vi "3-6For循环的使用(下).vi"() -> ()   [LabVIEW 2018]
panel:
  out "字符串":string
  # "找到10000内的完数。完数指一个数恰好等于它本身的因子之和，例如28=14+7+4+2+1，6=3+2+1。"
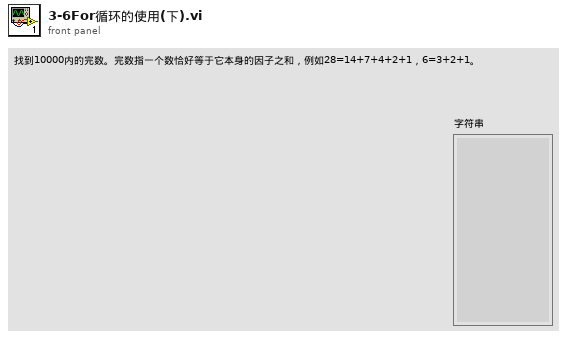
[diagram p1: front panel]
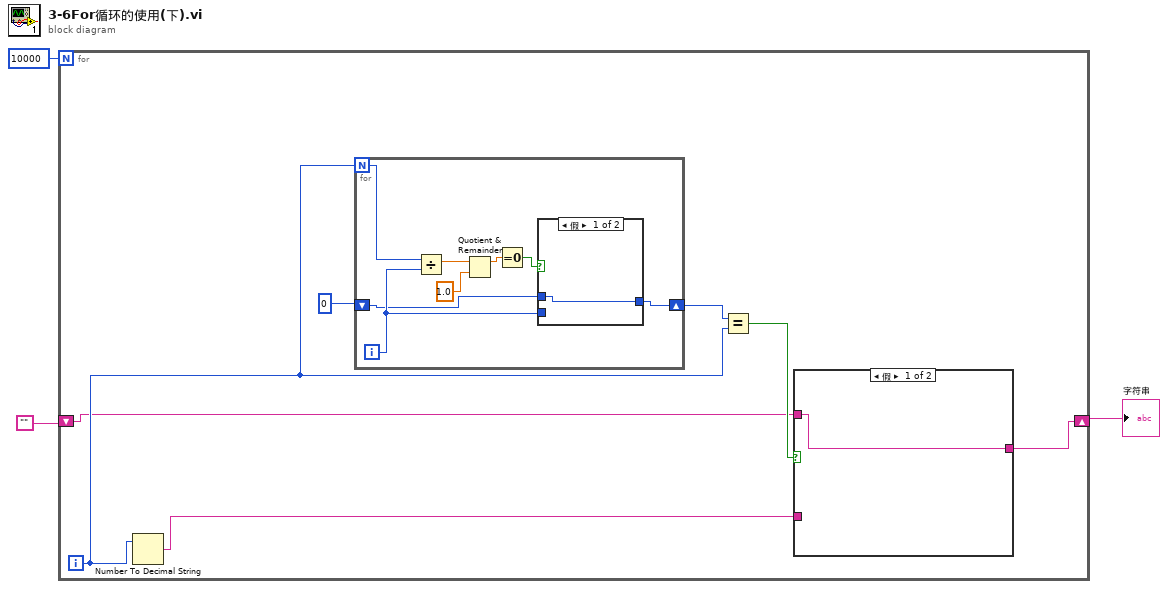
[diagram p0: block diagram]
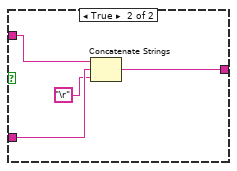
[diagram p2: hidden frame]
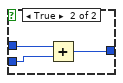
[diagram p3: hidden frame]
diagram:
  n1 = for {
    N: 10000 -> [_]
    shift-right: [w4] -> w1
    shift-left: "" -> [w6]
    i -> [w7]
    n2 = Number To Decimal String(number=w7) -> (decimal integer string=w5:string)  [unwired: 1 in]
    n3 = for {
      N: w7 -> [w23]
      shift-right: [w16] -> w9
      shift-left: 0 -> [w17]
      i -> [w18]
      n4 = Divide(x=w23, y=w18) -> (x/y=w22:dbl)
      n5 = Quotient & Remainder(x=w22, y=1.0) -> (x-y*floor(x/y)=w20:dbl)  [unwired: 1 out]
      n6 = Equal To 0?(x=w20) -> (x = 0?=w19:bool)
      n7 = case shown="假" w19 {
        tunnel: w18 -> [_ w27]
        tunnel: w17 -> [w24 w26]
        tunnel: [w24 w25] -> w16
        frame False {
        }
        frame True {
          n8 = Add(x=w26, y=w27) -> (x+y=w25:i32)
        }
      }
    }
    n9 = Equal?(x=w9, y=w7) -> (x = y?=w8:bool)
    n10 = case shown="假" w8 {
      tunnel: w6 -> [w11 w15]
      tunnel: w5 -> [_ w14]
      tunnel: [w11 w12] -> w4
      frame False {
      }
      frame True {
        n11 = Concatenate Strings(w15, w14, "\r") -> (w12:string)
      }
    }
  }
  "字符串" <- w1
